vi "Read Settings.vi"(8 "error in (no error)":errorcluster, 11 "Iterator Actor in":refnum<class "Iterator Actor.lvclass">) -> (0 "error out":errorcluster, 2 "Settings":T1={"Prepare timeout (ms)"=200, "Iterate timeout (ms)"=50, "Conclude timeout (ms)"=200, "Iterate period (ms)"=200, "Number of iterations"=5, "Stop Condition"=enum."None", "Time before stop (ms)"=5, "Prepare Msg"=refnum, "Iterate Msg"=refnum, "Conclude Msg"=refnum, "Error Handler"=refnum}, 3 "Iterator Actor out":refnum<class "Iterator Actor.lvclass">)   [LabVIEW 2016, in "Iterator Actor.lvlib" / "Iterator Actor.lvclass"]
doc: "Configures the parameters of the Iterator and starts the sequence."
uses:
  Iterator Actor.lvclass
  Iterator Settings.ctl
  Iterator Actor Abstract Messages/Iterator Reply Msg/Iterator Reply Msg.lvclass
  Iterator Actor Abstract Messages/Iterator Report Error Msg/Iterator Report Error Msg.lvclass
  Stop Condition.ctl
  Iterator Actor.lvclass/Iterator Actor.ctl
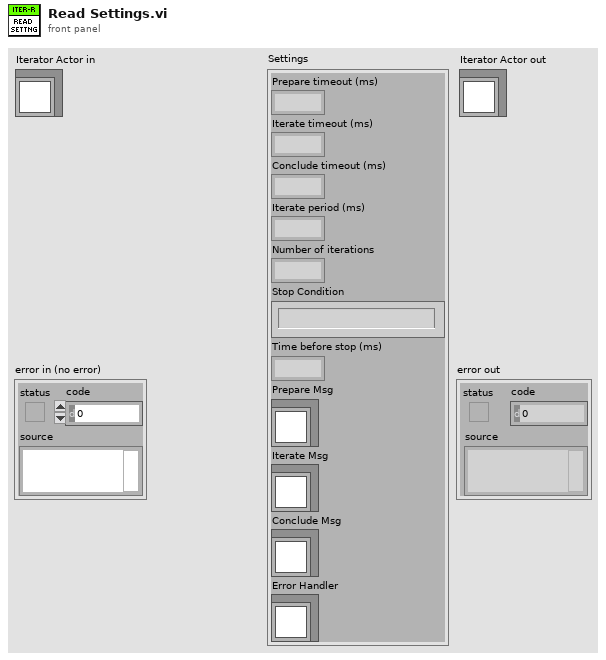
[diagram p1: front panel]
types:
  T1 = typedef "Iterator Actor.lvlib/Iterator Actor.lvclass/Iterator Settings.ctl" = cluster{"Prepare timeout (ms)":i32, "Iterate timeout (ms)":i32, "Conclude timeout (ms)":i32, "Iterate period (ms)":i32, "Number of iterations":i32, "Stop Condition":T2, "Time before stop (ms)":i32, "Prepare Msg":refnum<class "Iterator Reply Msg.lvclass">, "Iterate Msg":refnum<class "Iterator Reply Msg.lvclass">, "Conclude Msg":refnum<class "Iterator Reply Msg.lvclass">, "Error Handler":refnum<class "Iterator Report Error Msg.lvclass">}
  T2 = typedef "Iterator Actor.lvlib/Iterator Actor.lvclass/Stop Condition.ctl" = enum16{"None", "Number of iterations", "Time elapsed", "Iteration result"}
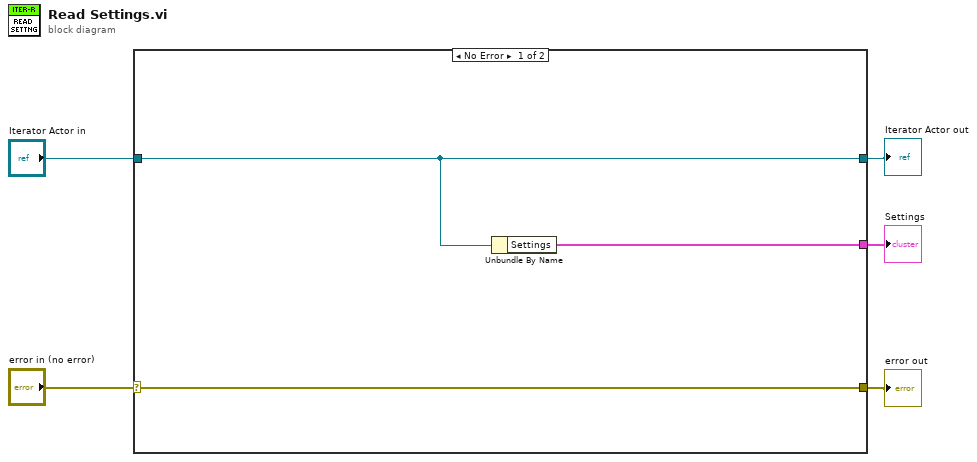
[diagram p0: block diagram]
diagram:
  n1 = case shown="No Error" "error in (no error)" {
    selector: "error in (no error)" -> [w8 w10]
    tunnel: [w8 w10] -> w4
    tunnel: [w7 w9] -> w2
    tunnel: "Iterator Actor in" -> [w7 w9]
    tunnel: [w6 _] -> w1
    frame No Error {
      n2 = Unbundle By Name(w7) -> ("Settings"=w6:T1)
    }
    frame Error {
    }
  }
  "error out" <- w4
  "Iterator Actor out" <- w2
  "Settings" <- w1
